vi "簇转成字符串.vi"(11 "起始点":cluster{"X":sgl, "Y":sgl}[](array[cluster])) -> (3 "字符串":string[](array[string]))   [LabVIEW 2017]
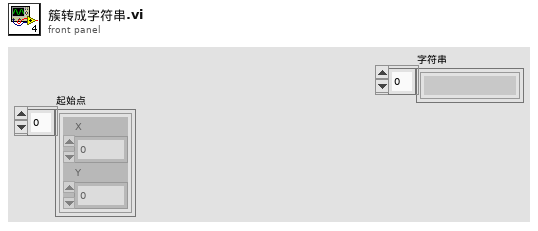
[diagram p1: front panel]
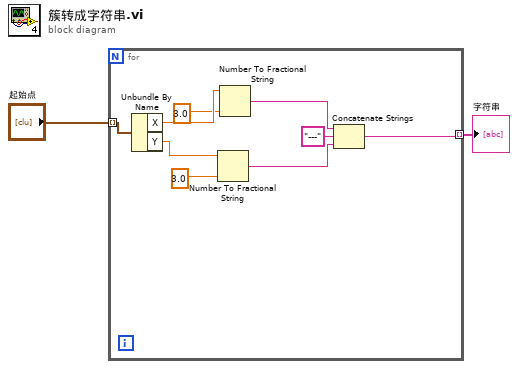
[diagram p0: block diagram]
diagram:
  n1 = for {
    tunnel: "起始点" -> [w11] mode=indexing
    tunnel: [w3] -> w1 mode=indexing
    n2 = Unbundle By Name(w11) -> ("X"=w10:sgl, "Y"=w8:sgl)
    n3 = Number To Fractional String(number=w8, precision (6)=sgl 3.0 ("X")) -> (F-format string=w4:string)  [unwired: 2 in]
    n4 = Number To Fractional String(number=w10, precision (6)=sgl 3.0 ("X")) -> (F-format string=w6:string)  [unwired: 2 in]
    n5 = Concatenate Strings(w6, "---" ("字符串"), w4) -> (w3:string)
  }
  "字符串" <- w1
